vi "VNA-ports to S-parameters.vi"(11 "VNA ports":bool[](array[boolean])=[TRUE, FALSE, FALSE, FALSE]) -> (1 "Sparameters (ports)":i32[][](array[numeric]), 2 "Sparameters (enum)":T1[](array[typedef]), 3 "Sparameters (string)":string[](array[string]), 5 "Number of ports":i32, 7 "Port numbers":i32[](array[numeric]))   [LabVIEW 2020]
uses:
  Instruments/Vector Network Analyzer/Controls/S parameter config control.ctl
  Instruments/Vector Network Analyzer/Vector Network Analyzer.lvclass
panel:
  out "Sparameter":T1=enum."Full 2 Port"
  out "Error Out":errorcluster
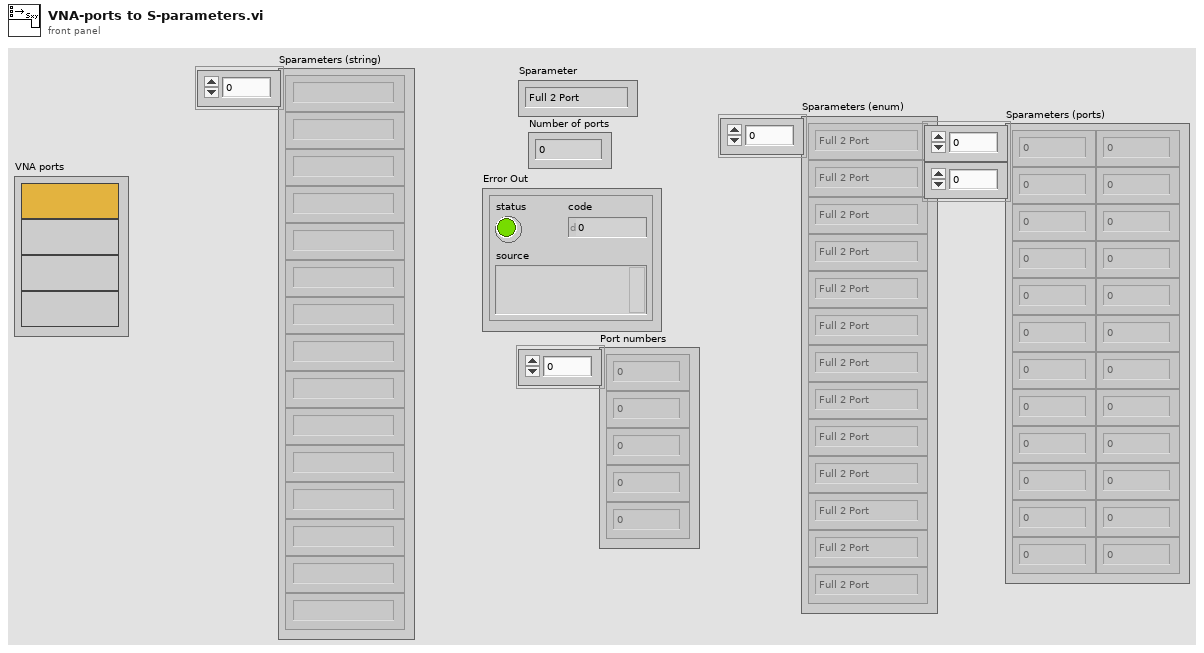
[diagram p1: front panel]
types:
  T1 = typedef "Vector Network Analyzer.lvclass/S parameter config control.ctl" = enum16{"S11", "S21", "S31", "S41", "S22", "S12", "S32", "S42", "S33", "S13", "S23", "S43", "S44", "S14", "S24", "S34", "Full 2 Port", "Full 3 Port", "Full 4 Port"}
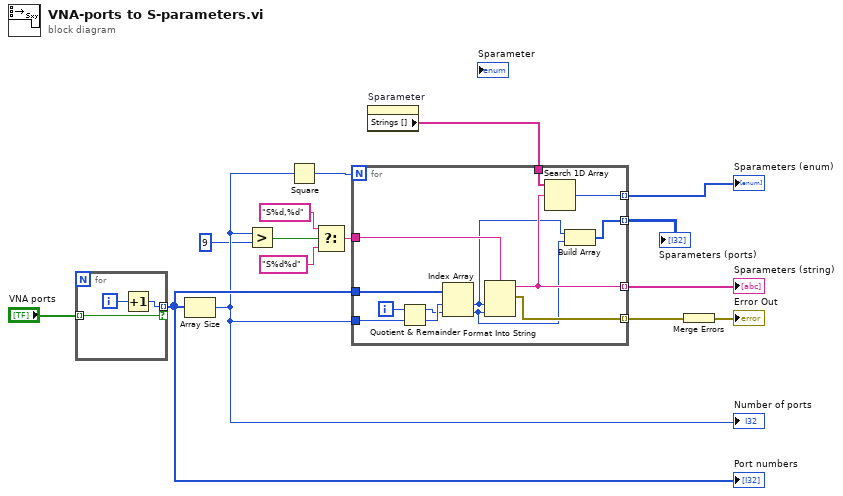
[diagram p0: block diagram]
diagram:
  n1 = for {
    tunnel: "VNA ports" -> [w18] mode=indexing
    tunnel: [w16] -> w12 mode=indexing if=w18
    i -> [w17]
    n2 = Increment(x=w17) -> (x+1=w16:i32)
  }
  "Port numbers" <- w12
  n3 = Array Size(array=w12) -> (size(s)=w7:i32)
  "Number of ports" <- w7
  n4 = Greater?(x=w7, y=9) -> (0:w5:bool)
  n5 = Square(x=w7) -> (x^2=w15:i32)
  n6 = Select(t="S%d,%d", s=w5, f="S%d%d") -> (s? t:f=w2:string)
  n7 = property on="Sparameter" class="Enum (strict)"() -> ("Strings []"=w9:string[])  [unwired: 2 in, 2 out]
  n8 = for {
    N: w15 -> [_]
    tunnel: w2 -> [w31]
    tunnel: [w23] -> w14 mode=indexing
    tunnel: w12 -> [w28]
    tunnel: w7 -> [w30]
    tunnel: [w25] -> w11 mode=indexing
    tunnel: w9 -> [w24]
    tunnel: [w22] -> w8 mode=indexing
    tunnel: [w19] -> w1 mode=indexing
    i -> [w29]
    n9 = Quotient & Remainder(x=w29, y=w30) -> (x-y*floor(x/y)=w26:i32, floor(x/y)=w27:i32)
    n10 = Index Array(array=w28, index #1=w27, index #2=w26) -> (element #1=w20:i32, element #2=w21:i32)
    n11 = Format Into String(format string=w31, w20, w21) -> (resulting string=w23:string, error out=w25:errorcluster)  [unwired: 2 in]
    n12 = Search 1D Array(1D array=w24, element=w23) -> (index of element=w22:i32)  [unwired: 1 in]
    n13 = Build Array(w20, w21) -> (w19:i32[])
  }
  "Sparameters (string)" <- w14
  "Sparameters (enum)" <- w8
  "Sparameters (ports)" <- w1
  n14 = Merge Errors(w11) -> (→"Error Out":errorcluster)
